vi "Get Message.vi"() -> (3 "Message":string="First Message")   [LabVIEW 2016]
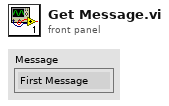
[diagram p1: front panel]
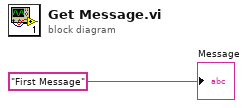
[diagram p0: block diagram]
diagram:
  "Message" <- "First Message"
